vi "Ej_EMA.vi"() -> ()   [LabVIEW 2020]
panel:
  out "Array":dbl[](array[numeric])
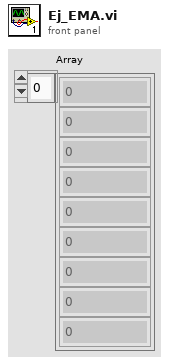
[diagram p1: front panel]
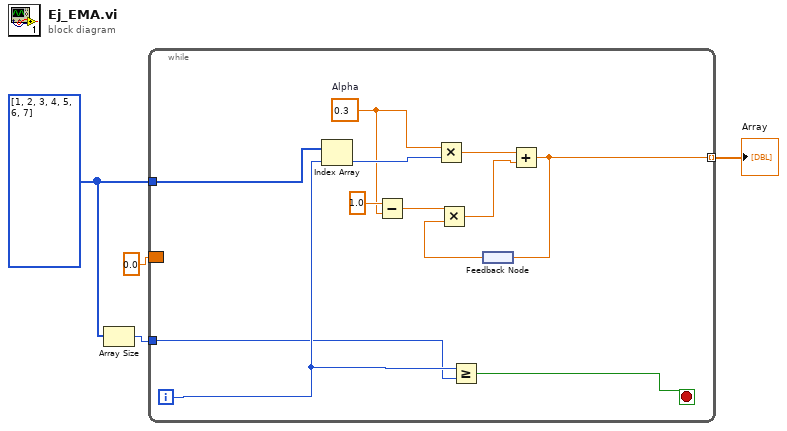
[diagram p0: block diagram]
diagram:
  w2 = i32[] [1, 2, 3, 4, 5, 6, 7]
  n1 = Array Size(array=w2) -> (size(s)=w1:i32)
  n2 = while {
    border: 0.0 -> [_]
    tunnel: [w9] -> w3 mode=indexing
    tunnel: w2 -> [w8]
    tunnel: w1 -> [w5]
    i -> [w7]
    stop <- w6 stop-if-true
    w12 = 0.3  # Alpha
    n3 = Index Array(array=w8, index=w7) -> (element=w14:i32)
    n4 = Subtract(x=1.0, y=w12) -> (x-y=w11:dbl)
    n5 = Multiply(x=w12, y=w14) -> (x*y=w15:dbl)
    n6 = Greater Or Equal?(x=w7, y=w5) -> (x >= y?=w6:bool)
    n7 = feedback #1() -> (w10:dbl)
    n8 = Multiply(x=w11, y=w10) -> (x*y=w16:dbl)
    n9 = Add(x=w15, y=w16) -> (x+y=w9:dbl)
    n10 = feedback-in #1(w9) -> ()
  }
  "Array" <- w3
